vi "PathPlanner_PathFinder_GetOpenNeighbors.vi"(11 "GridPosition S":T1) -> (3 "Open Neighbors":T1[](array[typedef]))   [LabVIEW 2019]
uses:
  PathPlannerLib24/TypeDef/PathPlannerFinderGridPosition.ctl
  PathPlannerLib24/VI/PathPlanner_PathFinder_Globals.vi
  PathPlannerLib24/PathPlanner24.lvlib
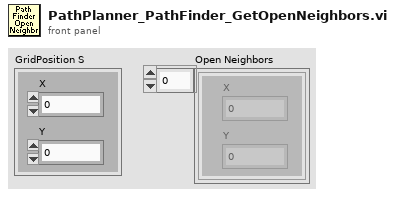
[diagram p1: front panel]
types:
  T1 = typedef "PathPlanner24.lvlib/PathPlannerFinderGridPosition.ctl" = cluster{"X":i32, "Y":i32}
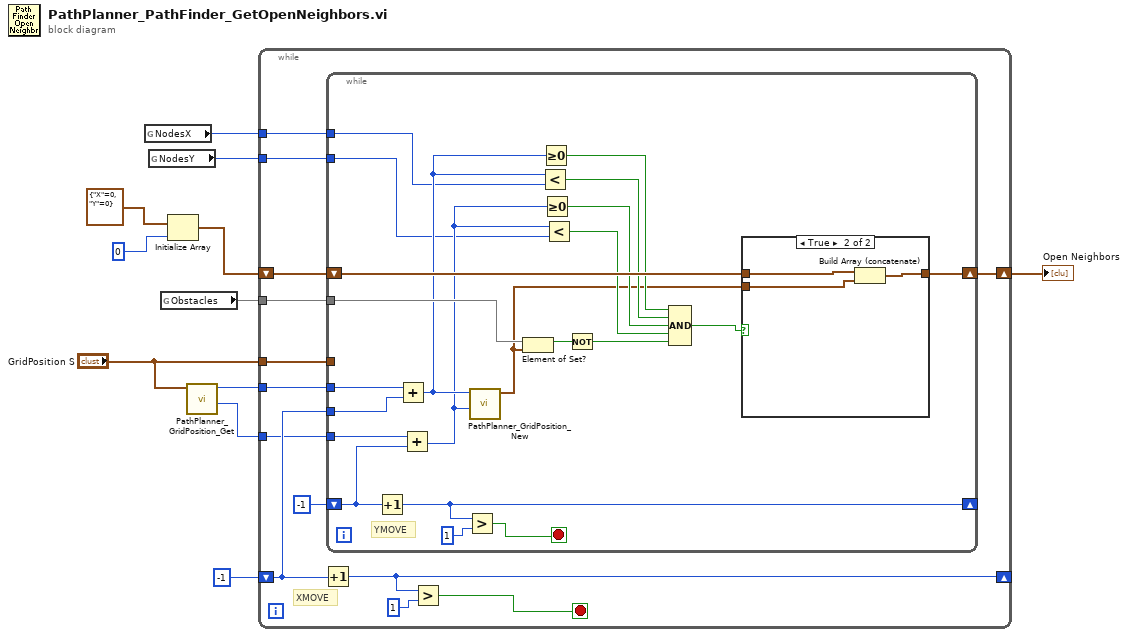
[diagram p0: block diagram]
diagram:
  n1 = global read "PathPlanner_PathFinder_Globals.vi" "NodesX"() -> (w2:i32)
  n2 = global read "PathPlanner_PathFinder_Globals.vi" "NodesY"() -> (w1:i32)
  n3 = global read "PathPlanner_PathFinder_Globals.vi" "Obstacles"() -> (w6:set{T1})
  n4 = Initialize Array(T1 {"X"=0, "Y"=0} ("Neighbors"), 0 ("dimension size")) -> (w5:T1[])
  n5 = call "PathPlanner_GridPosition_Get.vi"("GridPosition"="GridPosition S") -> ("Int Y"=w7:i32, "Int X"=w8:i32)  [unwired: 9 in]
  n6 = while {
    shift-right: [w24] -> _
    shift-left: -1 ("dimension size") -> [w20]
    tunnel: w8 -> [w19]
    tunnel: w7 -> [w18]
    tunnel: w6 -> [w17]
    shift-right: [w14] -> w3
    shift-left: w5 -> [w16]
    tunnel: "GridPosition S" -> [w15]
    tunnel: w2 -> [w13]
    tunnel: w1 -> [w12]
    stop <- w22 stop-if-true
    # "XMOVE"
    n7 = Increment(x=w20) -> (x+1=w24:i32)
    n8 = while {
      shift-right: [w44] -> _
      shift-left: -1 ("dimension size") -> [w41]
      tunnel: w20 -> [w43]
      tunnel: w19 -> [w42]
      tunnel: w18 -> [w40]
      tunnel: w17 -> [w37]
      shift-right: [w38] -> w14
      shift-left: w16 -> [w39]
      tunnel: w15 -> [_]
      tunnel: w13 -> [w32]
      tunnel: w12 -> [w31]
      stop <- w45 stop-if-true
      # "YMOVE"
      n9 = Increment(x=w41) -> (x+1=w44:i32)
      n10 = Add(x=w42, y=w43) -> (x+y=w34:i32)
      n11 = Add(x=w40, y=w41) -> (x+y=w33:i32)
      n12 = Greater?(x=w44, y=1) -> (0:w45:bool)
      n13 = call "PathPlanner_GridPosition_New.vi"("Int Y"=w33, "Int X"=w34) -> ("GridPosition"=w25:T1)  [unwired: 9 in]
      n14 = Element of Set?(10:w25, 11:w37) -> (3:w36:bool)
      n15 = Less?(x=w34, y=w32) -> (x < y?=w28:bool)
      n16 = Greater Or Equal To 0?(x=w34) -> (x >= 0?=w27:bool)
      n17 = Greater Or Equal To 0?(x=w33) -> (x >= 0?=w29:bool)
      n18 = Less?(x=w33, y=w31) -> (x < y?=w30:bool)
      n19 = Not(x=w36) -> (.not. x?=w35:bool)
      n20 = Compound Arithmetic op=AND(w27, w28, w29, w30, w35) -> (w26:bool)
      n21 = case shown="True" w26 {
        tunnel: w39 -> [w47 w50]
        tunnel: w25 -> [_ w49]
        tunnel: [w47 w48] -> w38
        frame False {
        }
        frame True {
          n22 = Build Array (concatenate)(w50, w49) -> (w48:T1[])
        }
      }
    }
    n23 = Greater?(x=w24, y=1) -> (0:w22:bool)
  }
  "Open Neighbors" <- w3
